vi "拉取dll.vi"(8 "error in (no error)":errorcluster, 11 "名称或相对路径":string="FreeMem.zip") -> (0 "error out":errorcluster)   [LabVIEW 2016, in "数据传输系统-03.lvlib" / "update.lvlib"]
uses:
  update.lvlib
  http client class/http client.lvclass
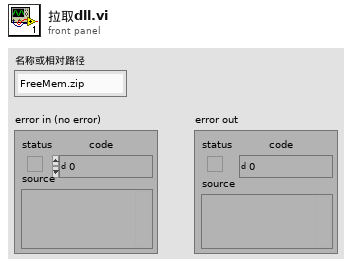
[diagram p1: front panel]
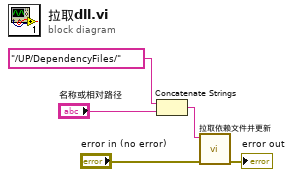
[diagram p0: block diagram]
diagram:
  n1 = Concatenate Strings("/UP/DependencyFiles/" ("远端地址"), "名称或相对路径") -> (w3:string)
  n2 = call "拉取依赖文件并更新.vi"("error in (no error)"="error in (no error)", "远端地址"=w3) -> ("error out"=→"error out":errorcluster)  [unwired: 9 in]
